vi "Dyno Data Converter.vi"(0 "VShunt":dbl, 1 "VGen":dbl) -> (2 "RPM":dbl, 3 "Torque":dbl, 4 "HP":dbl)   [LabVIEW 2014]
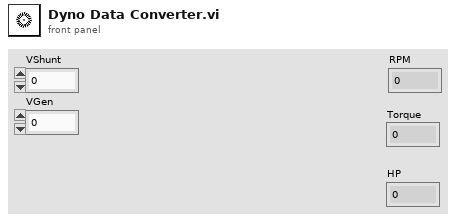
[diagram p1: front panel]
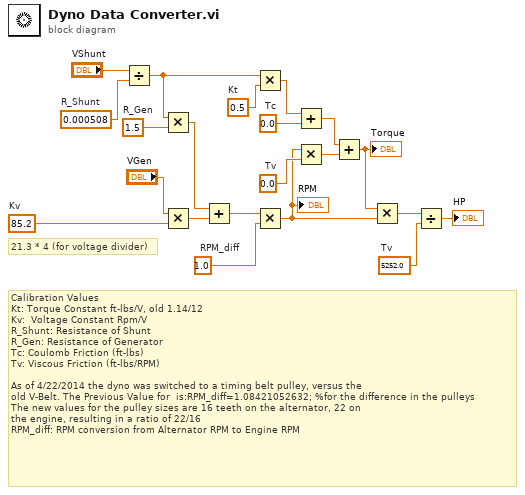
[diagram p0: block diagram]
diagram:
  w1 = 5252.0  # Tv
  w6 = 0.0  # Tv
  w10 = 0.0  # Tc
  w12 = 0.5  # Kt
  w15 = 1.0  # RPM_diff
  w16 = 85.2  # Kv
  w19 = 1.5  # R_Gen
  w20 = 0.000508  # R_Shunt
  # "Calibration Values\nKt: Torque Constant ft-lbs/V, old 1.14/12\nKv:  Voltage Constant Rpm/V\nR_Shunt: Resistance of Shunt\nR_Gen: Resistance of Generator\nTc: Coulomb Friction (ft-lbs)\nTv: Viscous Friction (ft-lbs/RPM)\n\nAs of 4/22/2014 the dyno was switched to a timing belt pulley, versus the\nold V-Belt. The Previous Value for  is:RPM_diff=1.08421052632; %for the difference in the pulleys\nThe new values for the pulley sizes are 16 teeth on the alternator, 22 on\nthe engine, resulting in a ratio of 22/16\nRPM_diff: RPM conversion from Alternator RPM to Engine RPM"
  # "21.3 * 4 (for voltage divider)"
  n1 = Divide(x="VShunt", y=w20) -> (x/y=w11:dbl)
  n2 = Multiply(x=w11, y=w19) -> (x*y=w14:dbl)
  n3 = Multiply(x="VGen", y=w16) -> (x*y=w18:dbl)
  n4 = Add(x=w14, y=w18) -> (x+y=w13:dbl)
  n5 = Multiply(x=w11, y=w12) -> (x*y=w9:dbl)
  n6 = Multiply(x=w13, y=w15) -> (x*y=w2:dbl)
  "RPM" <- w2
  n7 = Add(x=w9, y=w10) -> (x+y=w8:dbl)
  n8 = Multiply(x=w2, y=w6) -> (x*y=w7:dbl)
  n9 = Add(x=w8, y=w7) -> (x+y=w3:dbl)
  "Torque" <- w3
  n10 = Multiply(x=w3, y=w2) -> (x*y=w4:dbl)
  n11 = Divide(x=w4, y=w1) -> (x/y=→"HP":dbl)
